vi "Value Change.vi"(8 "error in (no error)":errorcluster, 9 "NewVal":i32[](array[numeric]), 10 "Debugger":refnum<class "Debug Process.lvclass">, 11 "List Processes View Model In":refnum<class "List Messages View Model.lvclass">) -> (0 "error out":errorcluster, 3 "List Processes View Model Out":refnum<class "List Messages View Model.lvclass">)   [LabVIEW 2020, in "List Messages View Model.lvclass"]
uses:
  List Messages View Model.lvclass
  List Messages View Model.lvclass/List Messages View Model.ctl
  Debugger/Debugger.lvclass
  List Box View Model_/List Box View Model.lvclass
  C:/Users/anton/Documents/GitHub/triarc-debugger/source/List Box View Model_/List Box View Model.lvclass
  C:/Users/anton/Documents/GitHub/triarc-debugger/source/List Seen Messages View Model/List Messages View Model.lvclass
  Process/Debug Process.lvclass
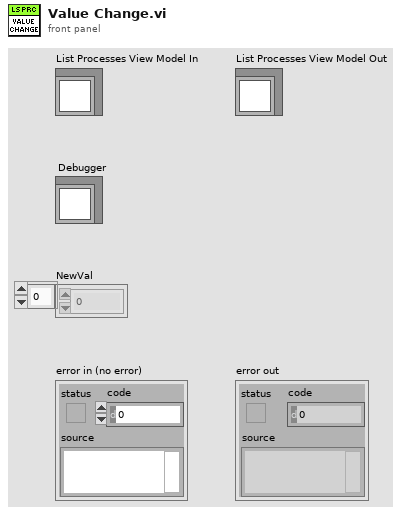
[diagram p1: front panel]
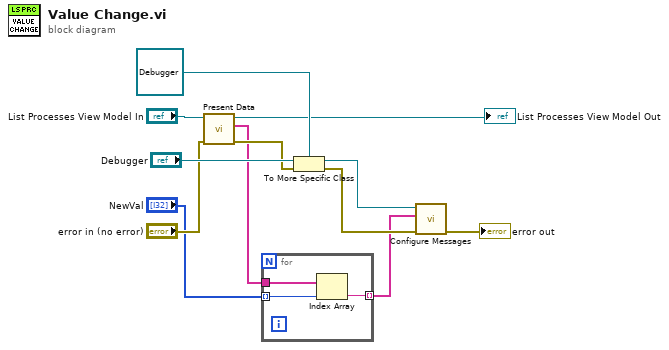
[diagram p0: block diagram]
diagram:
  n1 = call "Present Data.vi"("error in (no error)"="error in (no error)", "List Seen Processes View Model In"="List Processes View Model In") -> ("error out"=w6:errorcluster, "Message List"=w2:string[], "List Seen Processes View Model Out"=→"List Processes View Model Out":refnum<class "List Messages View Model.lvclass">)  [unwired: 7 in]
  n2 = for {
    tunnel: "NewVal" -> [w15] mode=indexing
    tunnel: w2 -> [w14]
    tunnel: [w13] -> w1 mode=indexing
    n3 = Index Array(array=w14, index=w15) -> (element=w13:string)
  }
  n4 = To More Specific Class(target class=refnum<class "Debugger.lvclass"> refnum ("Debugger.lvclass"), reference="Debugger", error in=w6) -> (specific class reference=w7:refnum<class "Debugger.lvclass">, error out=w10:errorcluster)
  n5 = call "Configure Messages.vi"("error in (no error)"=w10, "Messages"=w1, "Debugger In"=w7) -> ("error out"=→"error out":errorcluster)  [unwired: 7 in, 1 out]
